vi "Load Configuration Settings from XML.vi"(8 "error in (no error)":errorcluster, 11 "User Specified":T1={"Hardware Configuration"={"Signal Channel"="PXI1Slot7/ao0", "Response Channel"="PXI1Slot7/ai0", "Trigger Channel"="/PXI1Slot7/PFI0", "Number of Acquisitions"=1.0}, "Analysis Configuration"={"Statistics"=TRUE}, "Signal Type"=enum."From Excel", "New Data Behavior"=enum."Replace", "Signal Configuration"={"Chirp Amplitude"=0.0, "I/O Limit"=0.0, "Sample Rate"=0.0, "Chirp Duration (s)"=0.0, "Upper Frequency"=0.0, "Lower Frequency"=0.0, "Windowing"=enum."None"}, "Waveform File"="", "Save Location"=""}) -> (0 "error out":errorcluster, 3 "User Specified 2":T1={"Hardware Configuration"={"Signal Channel"="PXI1Slot7/ao0", "Response Channel"="PXI1Slot7/ai0", "Trigger Channel"="/PXI1Slot7/PFI0", "Number of Acquisitions"=1.0}, "Analysis Configuration"={"Statistics"=TRUE}, "Signal Type"=enum."From Excel", "New Data Behavior"=enum."Replace", "Signal Configuration"={"Chirp Amplitude"=0.0, "I/O Limit"=0.0, "Sample Rate"=0.0, "Chirp Duration (s)"=0.0, "Upper Frequency"=0.0, "Lower Frequency"=0.0, "Windowing"=enum."None"}, "Waveform File"="", "Save Location"=""})   [LabVIEW 2017]
doc: "Attempts to load previous user specified settings from an XML file.\n\nThis VI will not generate an error. If a suitable XML file can't be loaded and parsed then it will simply return the default settings."
uses:
  controls/User Specified Data.ctl
  controls/HW Configuration.ctl
  controls/Analysis Configuration.ctl
  controls/New Data Behavior.ctl
  controls/Signal Configuration.ctl
  <vilib>/Utility/xml.llb/Read From XML File(string).vi
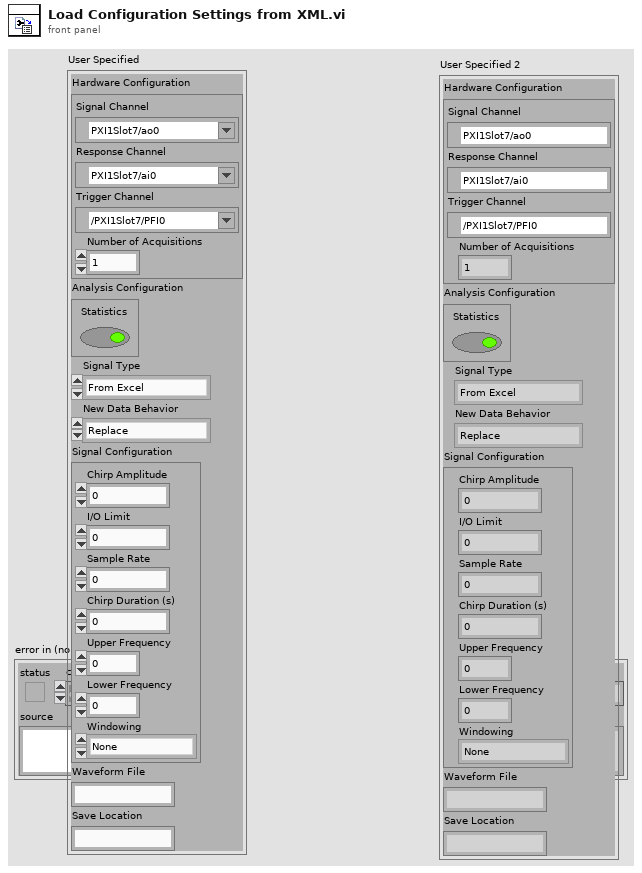
[diagram p1: front panel]
types:
  T1 = typedef "User Specified Data.ctl" = cluster{"Hardware Configuration":T2, "Analysis Configuration":T3, "Signal Type":enum16{"From Excel", "Single Chirp"}, "New Data Behavior":T4, "Signal Configuration":T5, "Waveform File":string, "Save Location":string}
  T2 = typedef "HW Configuration.ctl" = cluster{"Signal Channel":tag, "Response Channel":tag, "Trigger Channel":tag, "Number of Acquisitions":dbl}
  T3 = typedef "Analysis Configuration.ctl" = cluster{"Statistics":bool}
  T4 = typedef "New Data Behavior.ctl" = enum16{"Replace", "Overlay", "Append"}
  T5 = typedef "Signal Configuration.ctl" = cluster{"Chirp Amplitude":dbl, "I/O Limit":dbl, "Sample Rate":dbl, "Chirp Duration (s)":dbl, "Upper Frequency":dbl, "Lower Frequency":dbl, "Windowing":enum16{"None", "Exponential", "Flat top", "Hamming", "Hanning", "Kaiser-Bessel", "Rectangular"}}
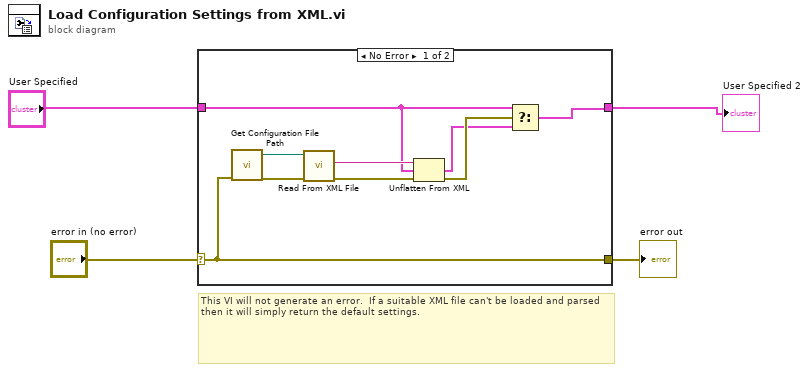
[diagram p0: block diagram]
diagram:
  # "This VI will not generate an error.  If a suitable XML file can't be loaded and parsed then it will simply return the default settings."
  n1 = case shown="No Error" "error in (no error)" {
    selector: "error in (no error)" -> [w10 w15]
    tunnel: [w10 w15] -> w3
    tunnel: "User Specified" -> [w7 w14]
    tunnel: [w5 w14] -> w1
    frame No Error {
      n2 = call "Get Configuration File Path.vi"("error in (no error)"=w10) -> ("error out"=w12:errorcluster, "XML File Path"=w13:path)  [unwired: 9 in]
      n3 = call-poly <vilib>:"Read From XML File.vi"("error in (no error)"=w12, "XML File Path"=w13) -> ("error out"=w9:errorcluster, "XML Elements"=w11:string)  [unwired: 7 in, 1 out]
      n4 = Unflatten From XML(xml string=w11, type=w7, error in (no error)=w9) -> (value=w6:T1, error out=w8:errorcluster)
      n5 = Select(t=w7, s=w8, f=w6) -> (s? t:f=w5:T1)
    }
    frame Error {
    }
  }
  "error out" <- w3
  "User Specified 2" <- w1
